vi "test-trajectory-transform-02.vi"() -> (3 "Test Passed":bool)   [LabVIEW 2019]
uses:
  <vilib>/Rock Robotics/WPI/ThirdParty/JAS_Junk/TrajLib/TRAJECTORY_SPLINE_TYPE_ENUM.ctl
  <vilib>/Rock Robotics/WPI/ThirdParty/JAS_Junk/TrajLib/Rotation2d_CreateAngle.vi
  <vilib>/Rock Robotics/WPI/ThirdParty/JAS_Junk/TrajLib/Translation2d_Equals.vi
  <vilib>/Rock Robotics/WPI/ThirdParty/JAS_Junk/TrajLib/Rotation2d_Equals.vi
  <vilib>/Rock Robotics/WPI/ThirdParty/JAS_Junk/TrajLib/Util_CalcDist.vi
  <vilib>/Rock Robotics/WPI/ThirdParty/JAS_Junk/TrajLib/Trajectory_Library.lvlib
panel:
  out "XY Graph":cluster{dbl[], dbl[]}[](graph)
  out "ShapeOkay":bool
  out "Starting Pose Okay":bool
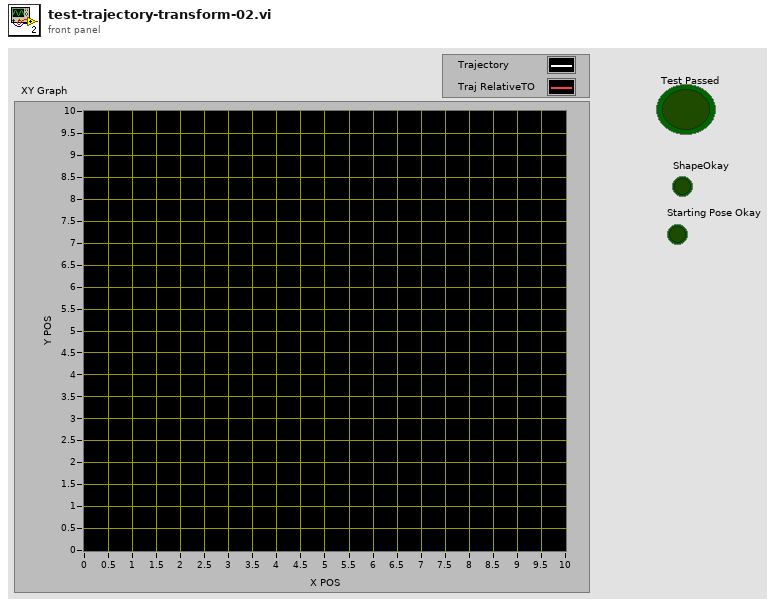
[diagram p1: front panel]
types:
  T1 = typedef "Trajectory_Library.lvlib/TRAJECTORY_SPLINE_TYPE_ENUM.ctl" = enum16{"Cubic", "Cubic With Weights", "Quintic", "Quintic With Weights"}
  T2 = typedef "Trajectory_Library.lvlib/WEIGHTED_WAYPOINT.ctl" = cluster{"TRANSLATION":T3, "ROTATION":T4, "SCALAR":dbl}
  T3 = typedef "Trajectory_Library.lvlib/TRANSLATION2D.ctl" = cluster{"X":dbl, "Y":dbl}
  T4 = typedef "Trajectory_Library.lvlib/ROTATION2D.ctl" = cluster{"VALUE":dbl, "COS":dbl, "SIN":dbl}
  T5 = typedef "Trajectory_Library.lvlib/TRAJ_CONFIG.ctl" = cluster{"MaxVelocity":dbl, "Max Acceleration":dbl, "StartVelocity":dbl, "End Velocity":dbl, "Reversed":bool, "DiffDrKineConstntDefined":bool, "CentAcellConstntDefined":bool, "DiffDrVoltConstntDefined":bool, "DIFF_DRIVE_KINE_CONSTRAINT":T6, "CENTRIPETAL_ACCEL_CONSTRAINT":T8, "SwerveDrKineConstntDefined":bool, "SWERVE_DRIVE_KINE_CONSTRAINT":T9, "DIFF_DRIVE_VOLTAGE_CONSTRAINT":T12, "MECANUM_DRIVE_KINE_CONSTRAINT":T14, "MecanumDrKineConstntDefined":bool}
  T6 = typedef "Trajectory_Library.lvlib/TRAJ_CONSTRAINT_DIIF_DRIVE_KINEMATICS.ctl" = cluster{"Max Speed (M/S)":dbl, "DIFF_DRIVE_KINEMATICS":T7, "Max Accel (M/S2)":dbl}
  T7 = typedef "Trajectory_Library.lvlib/DIFF_DRIVE_KINEMATICS.ctl" = cluster{"TrackWidth_Meters":dbl}
  T8 = typedef "Trajectory_Library.lvlib/TRAJ_CONSTRAINT_CENTRIPETAL_ACCEL.ctl" = cluster{"Max Cent Accel":dbl}
  T9 = typedef "Trajectory_Library.lvlib/TRAJ_CONSTRAINT_SWERVE_DRIVE_KINEMATICS.ctl" = cluster{"Max Speed (M/S)":dbl, "SwerveKinematics":T10}
  T10 = typedef "Trajectory_Library.lvlib/SWERVE_DRIVE_KINEMATICS.ctl" = cluster{"NumModules":i32, "InverseKinematics":T11, "ForwardKinematics":T11, "Modules":T3[], "PrevCoR":T3}
  T11 = typedef "NI_Matrix.lvlib/RealMatrix.ctl" = dbl[][]
  T12 = typedef "Trajectory_Library.lvlib/TRAJ_CONSTRAINT_DIIF_DRIVE_VOLTAGE.ctl" = cluster{"Max Voltage":dbl, "DIFF_DRIVE_KINEMATICS":T7, "SIMPLE_MOTOR_FF":T13}
  T13 = typedef "Trajectory_Library.lvlib/SIMPLE_MOTOR_FF.ctl" = cluster{"Ks":dbl, "Kv":dbl, "Ka":dbl}
  T14 = typedef "Trajectory_Library.lvlib/TRAJ_CONSTRAINT_MECA_DRIVE_KINEMATICS.ctl" = cluster{"Max Speed (M/S)":dbl, "MECA_DRIVE_KINEMATICS":T15}
  T15 = typedef "Trajectory_Library.lvlib/MECA_DRIVE_KINEMATICS.ctl" = cluster{"FrontLeft":T3, "FrontRight":T3, "RearLeft":T3, "RearRight":T3, "InverseKinematics":T11, "ForwardKinematics":T11, "PrevCoR":T3}
  T16 = typedef "Trajectory_Library.lvlib/TRAJECTORY.ctl" = cluster{"TotalTImeSecs":dbl, "States":T17[]}
  T17 = typedef "Trajectory_Library.lvlib/TRAJ_STATE.ctl" = cluster{"TimeSeconds":dbl, "Velocity":dbl, "Acceleration":dbl, "POSE":T18, "Curvature":dbl}
  T18 = typedef "Trajectory_Library.lvlib/POSE2D.ctl" = cluster{"TRANSLATION":T3, "ROTATION":T4}
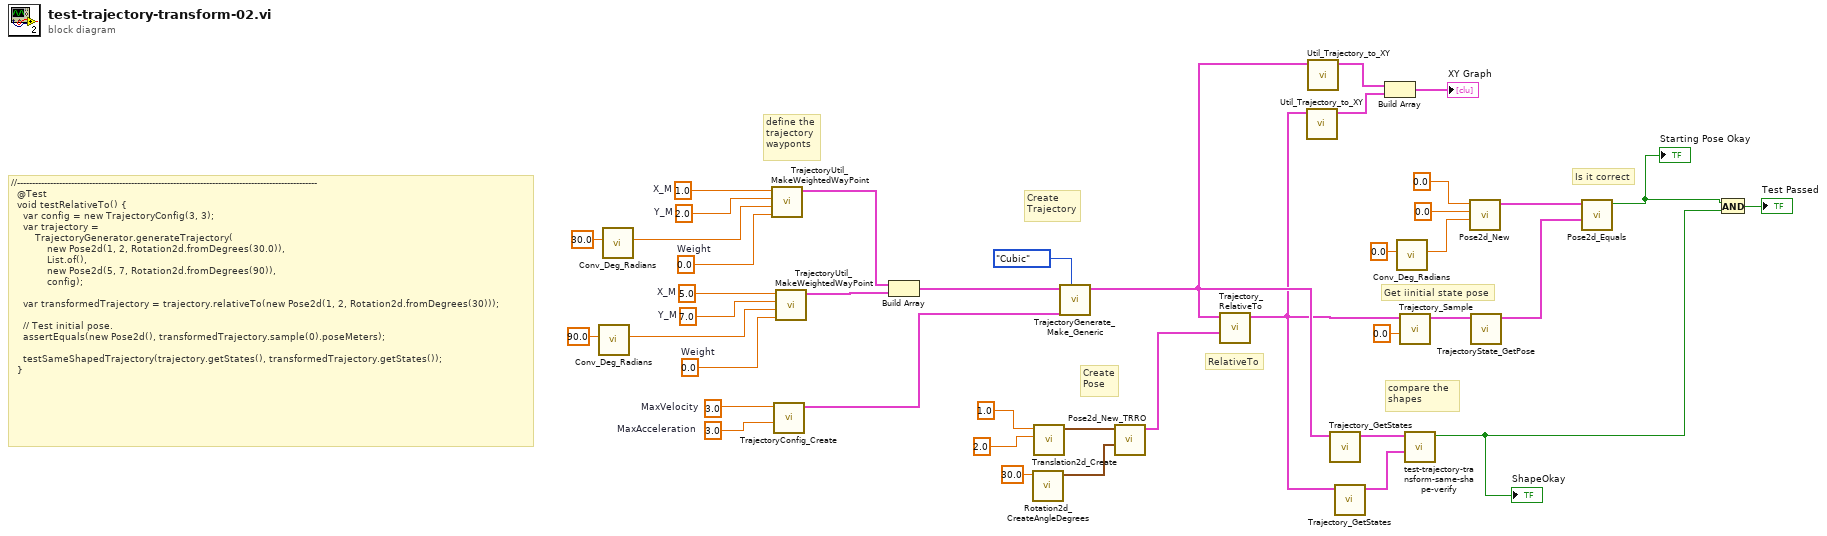
[diagram p0: block diagram]
diagram:
  w40 = 5.0  # X_M
  w39 = 7.0  # Y_M
  w38 = 0.0  # Weight
  w37 = 1.0  # X_M
  w36 = 2.0  # Y_M
  w35 = 0.0  # Weight
  w34 = 3.0  # MaxVelocity
  w33 = 3.0  # MaxAcceleration
  # "define the\ntrajectory\nwayponts"
  # "Is it correct"
  # "Get iinitial state pose"
  # "compare the \nshapes"
  # "RelativeTo"
  # "Create\nPose"
  # "Create\nTrajectory"
  # "//----------------------------------------------------------------------------------------------------\n  @Test\n  void testRelativeTo() {\n    var config = new TrajectoryConfig(3, 3);\n    var trajectory =\n        TrajectoryGenerator.generateTrajectory(\n            new Pose2d(1, 2, Rotation2d.fromDegrees(30.0)),\n            List.of(),\n            new Pose2d(5, 7, Rotation2d.fromDegrees(90)),\n            config);\n\n    var transformedTrajectory = trajectory.relativeTo(new Pose2d(1, 2, Rotation2d.fromDegrees(30)));\n\n    // Test initial pose.\n    assertEquals(new Pose2d(), transformedTrajectory.sample(0).poseMeters);\n\n    testSameShapedTrajectory(trajectory.getStates(), transformedTrajectory.getStates());\n  }"
  n1 = call <vilib>:"Conv_Deg_Radians.vi"("Degress"=90.0) -> ("Radians"=w27:dbl)  [unwired: 10 in]
  n2 = call <vilib>:"Conv_Deg_Radians.vi"("Degress"=30.0) -> ("Radians"=w9:dbl)  [unwired: 10 in]
  n3 = call <vilib>:"TrajectoryUtil_MakeWeightedWayPoint.vi"("Weight"=w35, "Travel Angle Radians"=w9, "Y_M"=w36, "X_M"=w37) -> ("WEIGHTED_WAYPOINT"=w29:T2)  [unwired: 7 in]
  n4 = call <vilib>:"TrajectoryConfig_Create.vi"("MaxAcceleration"=w33, "MaxVelocity"=w34) -> ("TRAJECTORY_CONFIG"=w32:T5)  [unwired: 9 in]
  n5 = call <vilib>:"TrajectoryUtil_MakeWeightedWayPoint.vi"("Weight"=w38, "Travel Angle Radians"=w27, "Y_M"=w39, "X_M"=w40) -> ("WEIGHTED_WAYPOINT"=w41:T2)  [unwired: 7 in]
  n6 = Build Array(w29, w41) -> (w30:T2[])
  n7 = call <vilib>:"Rotation2d_CreateAngleDegrees.vi"("Angle_Degrees"=30.0) -> ("ROTATION"=w7:T4)  [unwired: 10 in]
  n8 = call <vilib>:"Translation2d_Create.vi"("Y"=2.0, "X"=1.0) -> ("TRANSLATION"=w8:T3)  [unwired: 9 in]
  n9 = call <vilib>:"TrajectoryGenerate_Make_Generic.vi"("Spline Type"=TRAJECTORY_SPLINE_TYPE_ENUM."Cubic", "traj_config"=w32, "WeightedWayPoints"=w30) -> ("TRAJECTORY"=w5:T16)  [unwired: 7 in, 1 out]
  n10 = call <vilib>:"Pose2d_New_TRRO.vi"("ROTATION"=w7, "TRANSLATION"=w8) -> ("outPOSE"=w6:T18)  [unwired: 9 in]
  n11 = call <vilib>:"Trajectory_RelativeTo.vi"("POSE"=w6, "InputTRAJECTORY"=w5) -> ("outputTRAJECTORY"=w4:T16)  [unwired: 9 in]
  n12 = call <vilib>:"Util_Trajectory_to_XY.vi"("TRAJECTORY"=w4) -> ("outArrayXY"=w2:cluster{dbl[], dbl[]})  [unwired: 10 in]
  n13 = call <vilib>:"Util_Trajectory_to_XY.vi"("TRAJECTORY"=w5) -> ("outArrayXY"=w3:cluster{dbl[], dbl[]})  [unwired: 10 in]
  n14 = call <vilib>:"Trajectory_GetStates.vi"("TRAJECTORY"=w5) -> ("States"=w23:T17[])  [unwired: 10 in]
  n15 = call <vilib>:"Trajectory_GetStates.vi"("TRAJECTORY"=w4) -> ("States"=w22:T17[])  [unwired: 10 in]
  n16 = Build Array(w3, w2) -> (→"XY Graph":cluster{dbl[], dbl[]}[])
  n17 = call <vilib>:"Conv_Deg_Radians.vi"("Degress"=0.0) -> ("Radians"=w16:dbl)  [unwired: 10 in]
  n18 = call <vilib>:"Trajectory_Sample.vi"("Time"=0.0, "InputTRAJECTORY"=w4) -> ("OutputTRAJ_STATE"=w20:T17)  [unwired: 9 in]
  n19 = call "test-trajectory-transform-same-shape-verify.vi"("TrajStates2"=w22, "TrajStates1"=w23) -> ("SameShape"=w12:bool)  [unwired: 9 in]
  "ShapeOkay" <- w12
  n20 = call <vilib>:"Pose2d_New.vi"("Heading"=w16, "Y"=0.0, "X"=0.0) -> ("out POSe"=w15:T18)  [unwired: 8 in]
  n21 = call <vilib>:"TrajectoryState_GetPose.vi"("TRAJ_STATE"=w20) -> ("TrajStatePose"=w14:T18)  [unwired: 10 in]
  n22 = call <vilib>:"Pose2d_Equals.vi"("other POSE"=w14, "in POSE"=w15) -> ("Equals"=w13:bool)  [unwired: 9 in]
  "Starting Pose Okay" <- w13
  n23 = And(x=w13, y=w12) -> (x .and. y?=→"Test Passed":bool)
